vi "NI VeriStand - Set Channel Value by Data Reference.vi"(8 "error in (no error)":errorcluster, 10 "Value":dbl, 11 "Data Reference in":T1 format="%.0x") -> (0 "error out":errorcluster)   [LabVIEW 2020, in "Custom Device API.lvlib"]
doc: "Sets the value of the custom device channel specified by <B>Data Reference in</B>. Use the Get Channel Data Reference VI to get the channel data reference for this VI.\n\nYou can use this VI in the Execute Model case of an Inline Model Interface custom device, or in the Read Data from HW or Write Data to HW cases of an Inline Hardware Interface custom device. Do not use this VI outside of an inline custom device."
uses:
  <vilib>/NI VeriStand/Custom Device API/Custom Device API.lvlib
  <vilib>/NI VeriStand/Custom Device API/Data Reference.ctl
  <vilib>/NI VeriStand/Custom Device API/Global Data Refs.vi
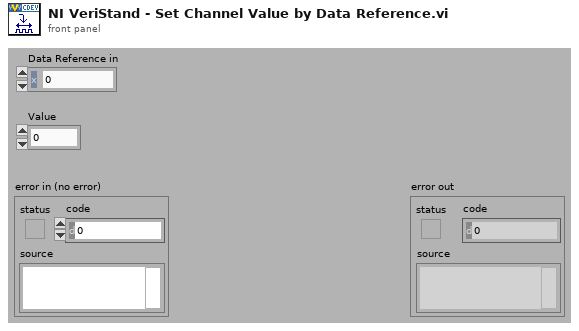
[diagram p1: front panel]
types:
  T1 = typedef "Custom Device API.lvlib/Data Reference.ctl" = i32
  T2 = typedef "Custom Device API.lvlib/Data Table Ref.ctl" = cluster{"Ptr.Beg":u64, "Ptr.End":u64}
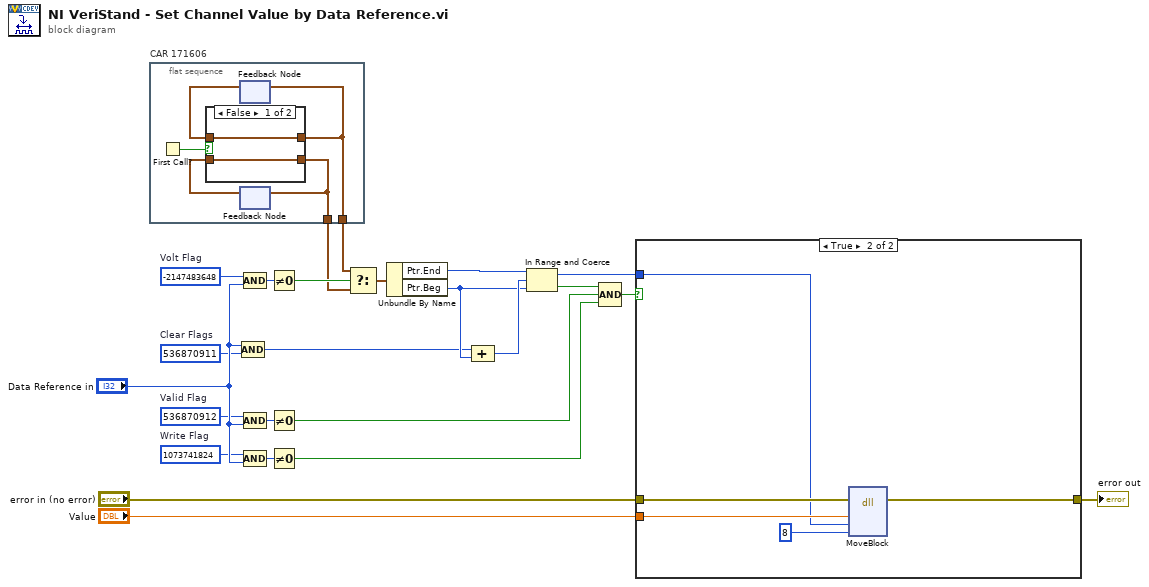
[diagram p0: block diagram]
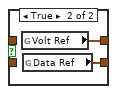
[diagram p2: hidden frame]
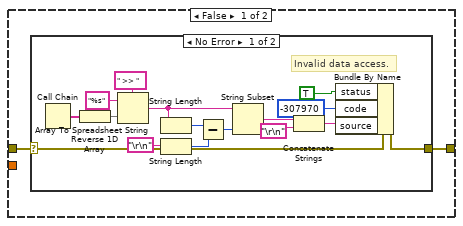
[diagram p3: hidden frame]
diagram:
  w4 = 536870911  # Clear Flags
  w7 = 1073741824  # Write Flag
  w13 = 536870912  # Valid Flag
  w11 = -2147483648  # Volt Flag
  n1 = flat-sequence "CAR 171606" {
    tunnel: [w27] -> w2
    tunnel: [w26] -> w1
    frame #0 {
      n2 = First Call?() -> (First Call?: T/F=w29:bool)
      n3 = feedback #1() -> (w28:T2)  [unwired: 1 out]
      n4 = feedback #2() -> (w25:T2)  [unwired: 1 out]
      n5 = case shown="False" w29 {
        tunnel: [w31 w33] -> w27
        tunnel: w28 -> [w31 _]
        tunnel: [w30 w32] -> w26
        tunnel: w25 -> [w30 _]
        frame False {
        }
        frame True {
          n6 = global read "Global Data Refs.vi" "Volt Ref"() -> (w33:T2)
          n7 = global read "Global Data Refs.vi" "Data Ref"() -> (w32:T2)
        }
      }
      n8 = feedback-in #1(w27) -> ()
      n9 = feedback-in #2(w26) -> ()
    }
  }
  n10 = Compound Arithmetic op=AND("Data Reference in", w4) -> (w3:T1)
  n11 = Compound Arithmetic op=AND(w11, "Data Reference in") -> (w10:T1)
  n12 = Compound Arithmetic op=AND(w13, "Data Reference in") -> (w14:T1)
  n13 = Compound Arithmetic op=AND(w7, "Data Reference in") -> (w6:T1)
  n14 = Not Equal To 0?(x=w10) -> (x != 0?=w12:bool)
  n15 = Not Equal To 0?(x=w14) -> (x != 0?=w8:bool)
  n16 = Not Equal To 0?(x=w6) -> (x != 0?=w5:bool)
  n17 = Select(t=w2, s=w12, f=w1) -> (s? t:f=w9:T2)
  n18 = Unbundle By Name(w9) -> ("Ptr.End"=w16:u64, "Ptr.Beg"=w19:u64)
  n19 = Compound Arithmetic op=ADD(w3, w19) -> (w20:u64)
  n20 = In Range and Coerce(upper limit=w16, x=w20, lower limit=w19) -> (coerced(x)=w18:u64, In Range?=w17:bool)
  n21 = Compound Arithmetic op=AND(w17, w8, w5) -> (w15:bool)
  n22 = case shown="True" w15 {
    tunnel: "error in (no error)" -> [w34 w57]
    tunnel: [w35 w53] -> w23
    tunnel: "Value" -> [_ w56]
    tunnel: w18 -> [_ w54]
    frame False {
      n23 = case shown="No Error" w34 {
        selector: w34 -> [w48 w52]
        tunnel: [w51 w52] -> w35
        frame No Error {
          # "Invalid data access."
          n24 = Call Chain() -> (call chain=w37:string[])
          n25 = Reverse 1D Array(array=w37) -> (reversed array=w44:string[])
          n26 = Array To Spreadsheet String(delimiter (Tab)=" >> ", array=w44, 3:"%s" ("format string")) -> (spreadsheet string=w45:string)
          n27 = String Length(string=w45) -> (length=w43:i32)
          n28 = String Length(string="\r\n") -> (length=w47:i32)
          n29 = Subtract(x=w43, y=w47) -> (x-y=w42:i32)
          n30 = String Subset(string=w45, length (rest)=w42) -> (substring=w38:string)  [unwired: 1 out]
          n31 = Concatenate Strings(w38, "\r\n") -> (w36:string)
          n32 = Bundle By Name(cluster=w48, "status"=TRUE, "code"=-307970, "source"=w36) -> (w51:errorcluster)
        }
        frame Error {
          # "Leave existing error."
        }
      }
    }
    frame True {
      n33 = dll-call lib="LabVIEW" fn="MoveBlock"(error in=w57, "ps"=w56, "pd"=w54, "size"=u64 8) -> (error out=w53:errorcluster)  [unwired: 5 in, 2 out]
    }
  }
  "error out" <- w23
